vi "main.vi"() -> ()   [LabVIEW 2017]
uses:
  Data Logger.lvclass
  C:/Program Files (x86)/National Instruments/LabVIEW 2017/vi.lib/ActorFramework/Actor/Actor.lvclass
  <vilib>/ActorFramework/Actor/Actor.lvclass
panel:
  in  "Boolean":bool
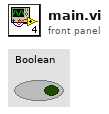
[diagram p1: front panel]
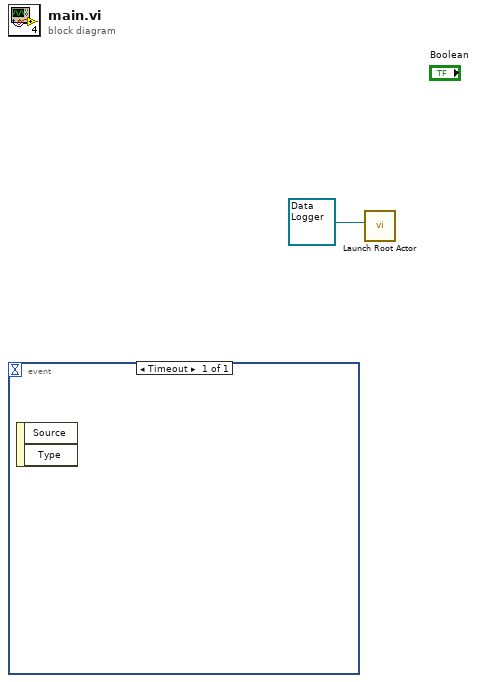
[diagram p0: block diagram]
diagram:
  n1 = event shown="[0] Timeout" {
    selector: _ -> [_]
    dyn-events: _ -> [_]
    timeout: _ -> [_]
    event Timeout {
      n2 = event-data() -> ()  [unwired: 1 in, 2 out]
    }
  }
  n3 = call <vilib>:"Launch Root Actor.vi"("Actor"=refnum<class "Data Logger.lvclass"> refnum ("Data Logger.lvlib:Data Logger.lvclass")) -> ()  [unwired: 9 in, 2 out]
